vi "Test Read Specific Type Tests.vi"() -> ()   [LabVIEW 2021]
uses:
  Source/Omni-Bus/Omni_Bus.lvclass
  Source/Aggregator Bus/Aggregator Bus.lvclass
  Source/Omni-Bus/Support/Broad Types.ctl
  <vilib>/TSA/Abstract Data Classes/Constants/Support/Str/Str.vi
  <vilib>/TSA/Abstract Data Classes/Constants/Support/Str/Const_Str.lvclass
  <vilib>/TSA/Abstract Data Classes/Constants/Support/DBL/DBL.vi
  <vilib>/TSA/Abstract Data Classes/Constants/Support/DBL/Const_DBL.lvclass
  <vilib>/TSA/Abstract Data Classes/Constants/Support/Bool/Bool.vi
  <vilib>/TSA/Abstract Data Classes/Constants/Support/Bool/Const_Bool.lvclass
  <vilib>/TSA/Abstract Data Classes/Constants/Support/U8/U8.vi
  <vilib>/TSA/Abstract Data Classes/Constants/Support/U8/Const_U8.lvclass
  <vilib>/TSA/Abstract Data Classes/Abs_Types/Boolean/Abs_Boolean.lvclass
  C:/Program Files (x86)/National Instruments/LabVIEW 2021/vi.lib/TSA/Abstract Data Classes/Abs_Types/Value/Abs_Value.lvclass
  C:/Program Files (x86)/National Instruments/LabVIEW 2021/vi.lib/TSA/Abstract Data Classes/Abs_Types/Type/Abs_Type.lvclass
  C:/Program Files (x86)/National Instruments/LabVIEW 2021/vi.lib/TSA/Abstract Data Classes/Abs_Types/Boolean/Abs_Boolean.lvclass
  C:/Program Files (x86)/National Instruments/LabVIEW 2021/vi.lib/TSA/Abstract Data Classes/Abs_Types/Double Float/Abs_Double Float.lvclass
  C:/Program Files (x86)/National Instruments/LabVIEW 2021/vi.lib/TSA/Abstract Data Classes/Abs_Types/Floating Point/Abs_Floating Point.lvclass
  C:/Program Files (x86)/National Instruments/LabVIEW 2021/vi.lib/TSA/Abstract Data Classes/Abs_Types/Numeric/Abs_Numeric.lvclass
  C:/Program Files (x86)/National Instruments/LabVIEW 2021/vi.lib/TSA/Abstract Data Classes/Constants/Support/DBL/Const_DBL.lvclass
  C:/Program Files (x86)/National Instruments/LabVIEW 2021/vi.lib/TSA/Abstract Data Classes/Constants/Support/Interface/Const_Intf.lvclass
  <vilib>/TSA/Abstract Data Classes/Abs_Types/String/Abs_String.lvclass
  C:/Program Files (x86)/National Instruments/LabVIEW 2021/vi.lib/TSA/Abstract Data Classes/Abs_Types/String/Abs_String.lvclass
  C:/Program Files (x86)/National Instruments/LabVIEW 2021/vi.lib/TSA/Abstract Data Classes/Abs_Types/U8 Integer/Abs_U8 Integer.lvclass
  C:/Program Files (x86)/National Instruments/LabVIEW 2021/vi.lib/TSA/Abstract Data Classes/Abs_Types/Integer/Abs_Integer.lvclass
  C:/Program Files (x86)/National Instruments/LabVIEW 2021/vi.lib/TSA/Abstract Data Classes/Constants/Support/U8/Const_U8.lvclass
  <vilib>/TSA/Abstract Data Classes/Abs_Types/Value/Abs_Value.lvclass
  C:/Users/Tim/Documents/GitHub/Omni-Bus/Source/Bus_Access/Bus_Access.lvclass
  C:/Users/Tim/Documents/GitHub/Omni-Bus/Source/Aggregator Bus/Aggregator Bus.lvclass
  <vilib>/TSA/Abstract Data Classes/Abs_Types/Double Float/Support/Type.ctl
  <vilib>/TSA/Abstract Data Classes/Abs_Types/Double Float/Abs_Double Float.lvclass
panel:
  in  "stop":bool
  out "Value":T1
  out "Tags":string[](array[string])
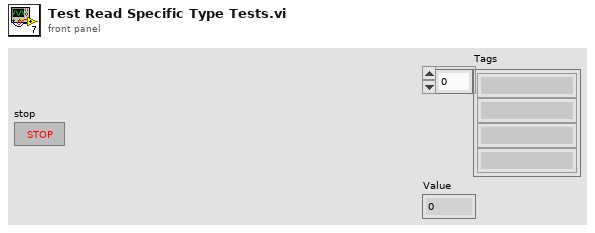
[diagram p1: front panel]
types:
  T1 = typedef "Abs_Double Float.lvclass/Type.ctl" = dbl
  T2 = typedef "Omni_Bus.lvclass/Broad Types.ctl" = enum16{"All Tags", "NI Specific Type", "Boolean", "String", "Numeric", "Float", "Integer", "Collection", "All Value Types", "Non Value Types"}
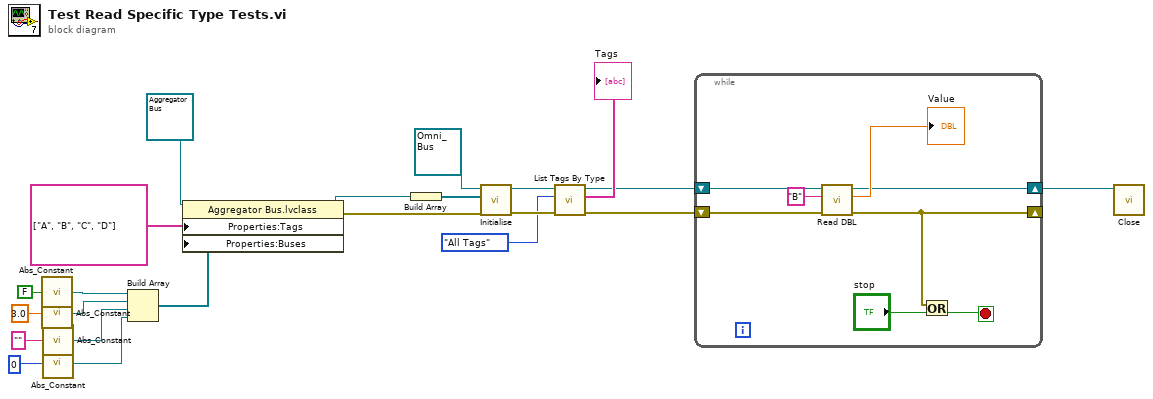
[diagram p0: block diagram]
diagram:
  n1 = call-poly <vilib>:"Abs_Constant.vi"("Boolean"=FALSE) -> ("Abs_Boolean.lvclass"=w16:refnum<class "Abs_Boolean.lvclass">)  [unwired: 4 in]
  n2 = call-poly <vilib>:"Abs_Constant.vi"("Value"=3.0) -> ("Constant"=w15:refnum<class "Const_DBL.lvclass">)  [unwired: 4 in]
  n3 = call-poly <vilib>:"Abs_Constant.vi"("String"="") -> ("Abs_String.lvclass"=w14:refnum<class "Abs_String.lvclass">)  [unwired: 4 in]
  n4 = call-poly <vilib>:"Abs_Constant.vi"("Value"=u8 0) -> ("Constant"=w6:refnum<class "Const_U8.lvclass">)  [unwired: 4 in]
  n5 = Build Array(w16, w15, w14, w6) -> (w11:refnum<class "Abs_Value.lvclass">[])
  n6 = property class="Aggregator Bus.lvclass"(reference=refnum<class "Aggregator Bus.lvclass"> refnum ("Data in"), "Properties:Tags"=string[] ["A", "B", "C", "D"] ("Tags"), "Properties:Buses"=w11) -> (reference out=w19:refnum<class "Aggregator Bus.lvclass">, error out=w20:errorcluster)  [unwired: 1 in]
  n7 = Build Array(w19) -> (w21:refnum<class "Aggregator Bus.lvclass">[])
  n8 = call-dynamic "Initialise.vi"("error in (no error)"=w20, "Bus Access"=w21, "Var Bus in"=refnum<class "Omni_Bus.lvclass"> refnum) -> ("error out"=w9:errorcluster, "Var Bus out"=w10:refnum<class "Omni_Bus.lvclass">)  [unwired: 7 in]
  n9 = call-dynamic "List Tags By Type.vi"("error in (no error)"=w9, "Broad Types"=Broad_Types."All Tags", "Var Bus in"=w10) -> ("error out"=w1:errorcluster, "Tags"=→"Tags":string[], "Var Bus out"=w2:refnum<class "Omni_Bus.lvclass">)  [unwired: 5 in, 1 out]
  n10 = while {
    shift-right: [w25] -> w3
    shift-left: w2 -> [w29]
    shift-right: [w23] -> _
    shift-left: w1 -> [w28]
    stop <- w24 stop-if-true
    n11 = call "Read DBL.vi"("error in (no error)"=w28, "Tag"="B", "Var Bus in"=w29) -> ("error out"=w23:errorcluster, "Numeric"=→"Value":dbl, "Var Bus out"=w25:refnum<class "Omni_Bus.lvclass">)  [unwired: 6 in]
    n12 = Or(x=w23, y="stop") -> (x .or. y?=w24:bool)
  }
  n13 = call-dynamic "Close.vi"("Data in"=w3) -> ()  [unwired: 9 in, 2 out]
